vi "getDACLimits.vi"(8 "error in":T1, 11 "DAC":T3 items=["DAC 1", "DAC 2", "DAC 3", "DAC 4"]) -> (0 "error out":T1, 3 "DAC-Limits out":T2={"Current Limit"=-inf, "LT-Limit"=-inf, "RT-Limit"=-inf} {"RT-Limit" format="%#_g V"; "LT-Limit" format="%#_g V"; "Current Limit" format="%#_g V"})   [LabVIEW 2016]
doc: "Reads out the DAC-Limits for a DAC defined by the input \"DAC\".\nThe ouput Cluster contains the following parameters\n -RT-Limit: set limit value for room temperature\n -LT-Limit: set limit value for low temperature\n -Current Limit: limit value as a result of interpolation regarding the current temperature."
uses:
  Controls/DAC_Selection.ctl
  Controls/DAC_Limits.ctl
  Controls/Error_Out.ctl
  Files_ASC500/DLL/ASC500_RemoteControlV27.dll
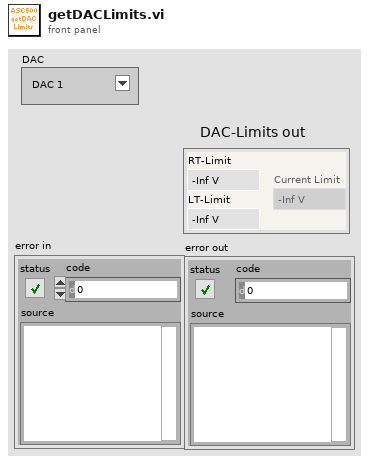
[diagram p1: front panel]
types:
  T1 = typedef "Error_Out.ctl" = errorcluster
  T2 = typedef "DAC_Limits.ctl" = cluster{"Current Limit":sgl, "LT-Limit":sgl, "RT-Limit":sgl}
  T3 = typedef "DAC_Selection.ctl" = u16
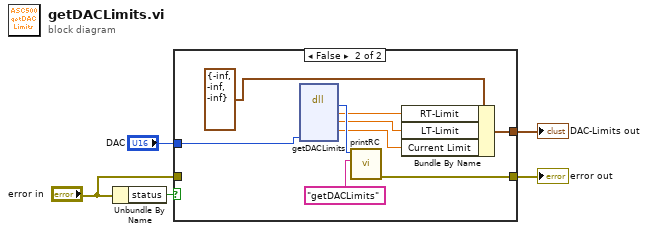
[diagram p0: block diagram]
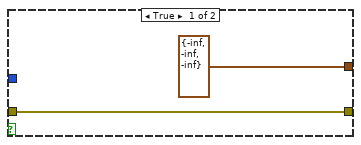
[diagram p2: hidden frame]
diagram:
  n1 = Unbundle By Name("error in") -> ("status"=w3:bool)
  n2 = case shown="False" w3 {
    tunnel: [w7 w15] -> w2
    tunnel: "error in" -> [w7 _]
    tunnel: [T2 {"Current Limit"=-inf, "LT-Limit"=-inf, "RT-Limit"=-inf} ("DAC-Limits out 2") w10] -> w4
    tunnel: "DAC" -> [_ w9]
    frame True {
    }
    frame False {
      n3 = dll-call lib="G:/SCMOperations/Share/ELE/Produkt Information/ASC500/04 Remote Control/02 development versions/2018Nov06/Files_ASC500/DLL/ASC500_RemoteControlV27.dll" fn="getDACLimits"("DAC"=w9) -> ("return type"=w16:i32, "RTLimit"=w13:sgl, "LTLimit"=w12:sgl, "CurrentDACLimit"=w11:sgl)  [unwired: 7 in, 2 out]
      n4 = call "printRC.vi"("additional information"="getDACLimits", "RC"=w16) -> ("error out"=w15:T1)  [unwired: 9 in]
      n5 = Bundle By Name(cluster=T2 {"Current Limit"=-inf, "LT-Limit"=-inf, "RT-Limit"=-inf} ("DAC-Limits out"), "RT-Limit"=w13, "LT-Limit"=w12, "Current Limit"=w11) -> (w10:T2)
    }
  }
  "error out" <- w2
  "DAC-Limits out" <- w4
